vi "Initialize Hardware References.vi"(8 "error in (no error)":errorcluster, 11 "Hardware Resources in":T1={"DO"={"task name"="AI", "task_ref"="", "lines"=""}}) -> (0 "error out":errorcluster, 3 "Hardware Resources out":T1={"DO"={"task name"="AI", "task_ref"="", "lines"=""}})   [LabVIEW 2014, in "PLS Digital Control.lvlib"]
doc: "Initialize the hardware references."
uses:
  PLS Digital Control.lvlib
  Hardware Configuration.ctl
  <vilib>/DAQmx/create/channels.llb/DAQmx Create Channel (DO-Digital Output).vi
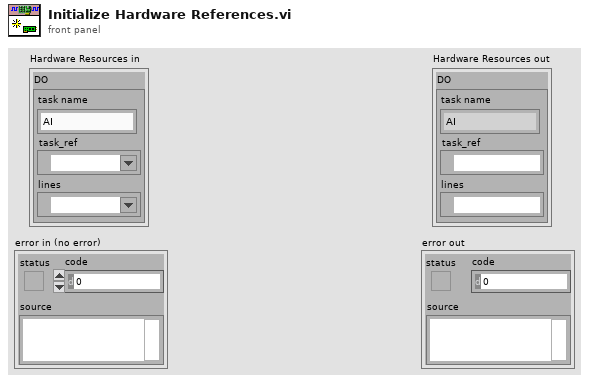
[diagram p1: front panel]
types:
  T1 = typedef "PLS Digital Control.lvlib/Hardware Configuration.ctl" = cluster{"DO":cluster{"task name":string, "task_ref":refnum<k21>, "lines":tag}}
  T2 = cluster{"task name":string, "task_ref":refnum<k21>, "lines":tag}
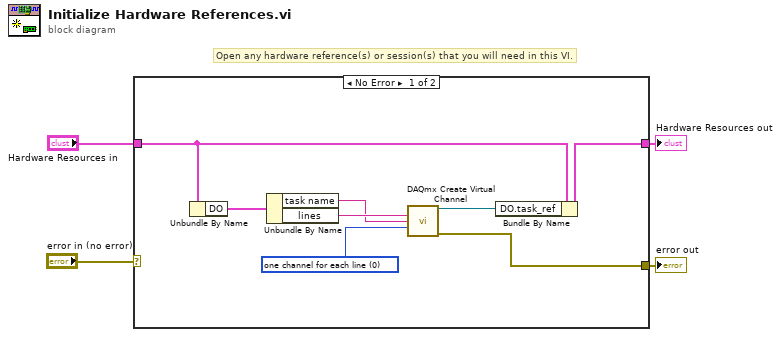
[diagram p0: block diagram]
diagram:
  # "Open any hardware reference(s) or session(s) that you will need in this VI."
  n1 = case shown="No Error" "error in (no error)" {
    selector: "error in (no error)" -> [_ w13]
    tunnel: [w5 w13] -> w3
    tunnel: "Hardware Resources in" -> [w8 w14]
    tunnel: [w7 w14] -> w1
    frame No Error {
      w11 = 0 items=["one channel for each line", "one channel for all lines"] ("line grouping")
      n2 = Unbundle By Name(w8) -> ("DO"=w9:T2)
      n3 = Unbundle By Name(w9) -> ("task name"=w10:string, "lines"=w12:tag)
      n4 = call-poly <vilib>:"DAQmx Create Virtual Channel.vi"("lines"=w12, "name to assign"=w10, "line grouping"=w11) -> ("task out"=w6:refnum<k21>, "error out"=w5:errorcluster)  [unwired: 11 in]
      n5 = Bundle By Name(cluster=w8, "DO.task_ref"=w6) -> (w7:T1)
    }
    frame Error {
    }
  }
  "Hardware Resources out" <- w1
  "error out" <- w3
